vi "Home Filter Wheel.vi"(8 "error in (no error)":errorcluster, 10 "Motor":i32, 11 "Filter Wheel Simulator in":refnum<class "Filter Wheel Simulator.lvclass">) -> (0 "error out":errorcluster, 1 "Success":bool, 2 "Log":string, 3 "Filter Wheel Simulator out":refnum<class "Filter Wheel Simulator.lvclass">)   [LabVIEW 2021, in "Filter Wheel Simulator.lvclass"]
uses:
  Filter Wheel Simulator.lvclass
  C:/Development/prime/Prime-RIMAS/Filter Wheel/Filter Wheel Object/Filter Wheel.lvclass
  Filter Wheel Object/Filter Wheel.lvclass
  Filter Wheel Simulator.lvclass/Filter Wheel Simulator.ctl
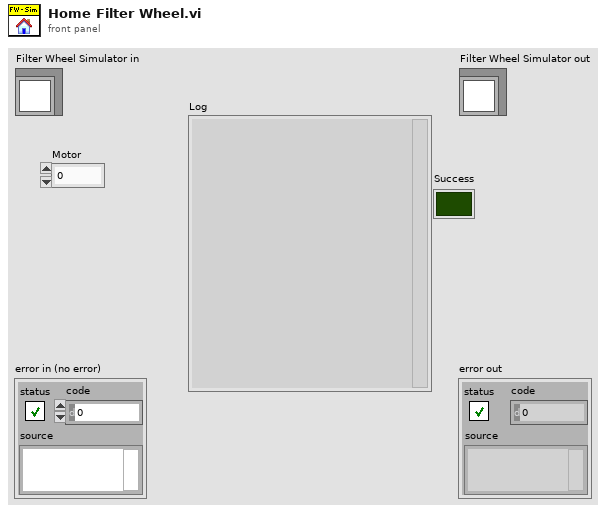
[diagram p1: front panel]
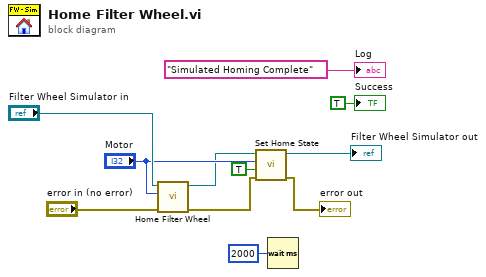
[diagram p0: block diagram]
diagram:
  n1 = call-parent "Home Filter Wheel.vi"("error in (no error)"="error in (no error)", "Motor"="Motor", "Filter Wheel in"="Filter Wheel Simulator in") -> ("error out"=w7:errorcluster, "Filter Wheel out"=w3:refnum<class "Filter Wheel Simulator.lvclass">)  [unwired: 5 in, 2 out]
  n2 = call "Set Home State.vi"("error in (no error)"=w7, "Home?"=TRUE, "Motor"="Motor", "Filter Wheel in"=w3) -> ("error out"=→"error out":errorcluster, "Filter Wheel out"=→"Filter Wheel Simulator out":refnum<class "Filter Wheel Simulator.lvclass">)  [unwired: 6 in]
  n3 = Wait (ms)(milliseconds to wait=u32 2000) -> ()  [unwired: 1 out]
  "Log" <- "Simulated Homing Complete"
  "Success" <- TRUE ("Success")
